vi "nettest.vi"() -> ()   [LabVIEW 2024]
uses:
  <vilib>/Utility/tcp.llb/UDP Multicast Read-Write Open.vi
panel:
  out "data out":string
  out "value":T1(array[cluster])
  out "port":u16
  out "address":u32
  out "current time":timestamp
  out "error out":errorcluster
  out "Numeric":i32
  in  "stop":bool
  out "length":i32
  out "data string":string
  in  "Array":dbl[](array[numeric])
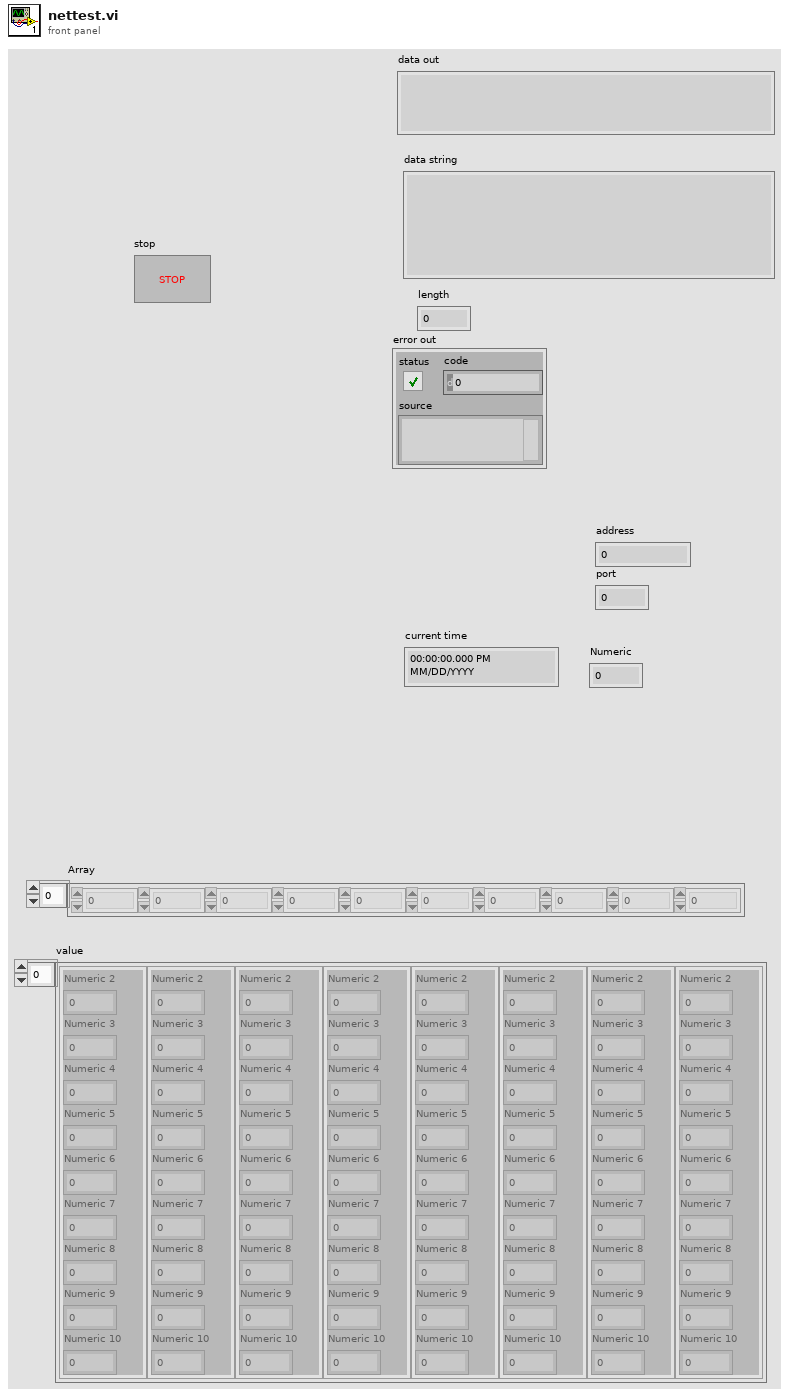
[diagram p1: front panel]
types:
  T1 = cluster{"Numeric 2":dbl, "Numeric 3":dbl, "Numeric 4":dbl, "Numeric 5":dbl, "Numeric 6":dbl, "Numeric 7":dbl, "Numeric 8":dbl, "Numeric 9":dbl, "Numeric 10":dbl}[]
  T2 = cluster{"Numeric 2":i16, "Numeric 3":i16, "Numeric 4":i16, "Numeric 5":i16, "Numeric 6":i16, "Numeric 7":i16, "Numeric 8":i16, "Numeric 9":i16, "Numeric 10":i16}[]
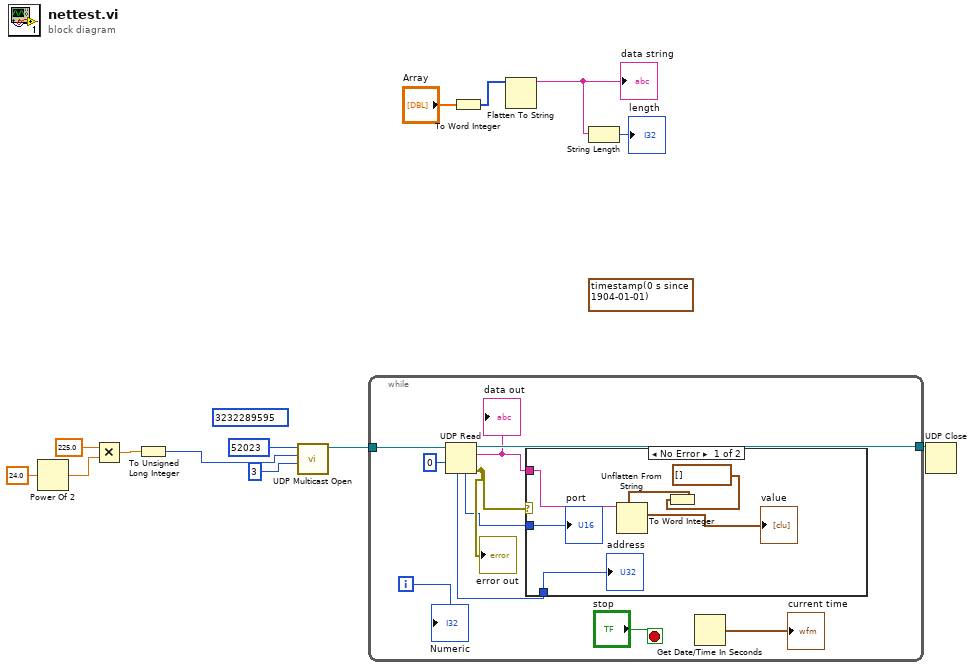
[diagram p0: block diagram]
diagram:
  (unwired) timestamp(0 s since 1904-01-01)
  (unwired) u32 3232289595 ("net address")
  n1 = Power Of 2(x=24.0) -> (2^x=w5:dbl)
  n2 = Multiply(x=225.0, y=w5) -> (x*y=w8:dbl)
  n3 = To Unsigned Long Integer(number=w8) -> (unsigned 32bit integer=w7:u32)
  n4 = call-poly <vilib>:"UDP Multicast Open.vi"("time-to-live (1)"=u16 3, "multicast addr"=w7, "port"=u16 52023) -> ("connection ID"=w11:refnum<k16>)  [unwired: 6 in, 2 out]
  n5 = while {
    tunnel: w11 -> [w23]
    tunnel: [w22] -> w10
    i -> [w19]
    stop <- "stop" stop-if-true
    n6 = UDP Read(connection ID=w23, timeout ms (25000)=0) -> (data out=w17:string, error out=w18:errorcluster, 3:w22:refnum<k16>, 4:w15:u16, 6:w14:u32)  [unwired: 2 in]
    "error out" <- w18
    "data out" <- w17
    n7 = case shown="No Error" w18 {
      tunnel: w17 -> [w29 _]
      tunnel: w15 -> [w28 _]
      tunnel: w14 -> [w27 _]
      frame No Error {
        n8 = To Word Integer(number=T1 [] ("Array")) -> (16bit integer=w25:T2)
        n9 = Unflatten From String(type=w25, binary string=w29) -> (value=→"value":T2)  [unwired: 3 in, 2 out]
        "port" <- w28
        "address" <- w27
      }
      frame Error {
      }
    }
    n10 = Get Date/Time In Seconds() -> (seconds since 1Jan1904=→"current time":timestamp)
    "Numeric" <- w19
  }
  n11 = To Word Integer(number="Array") -> (16bit integer=w1:i16[])
  n12 = Flatten To String(anything=w1) -> (data string=w13:string)  [unwired: 3 in, 2 out]
  "data string" <- w13
  n13 = String Length(string=w13) -> (length=→"length":i32)
  n14 = UDP Close(connection ID=w10) -> ()  [unwired: 1 in, 2 out]
